vi "Read was run.vi"(8 "error in (no error)":errorcluster, 11 "WasRun in":refnum<class "WasRun.lvclass">) -> (0 "error out":errorcluster, 2 "was run":bool, 3 "WasRun out":refnum<class "WasRun.lvclass">)   [LabVIEW 2013, in "WasRun.lvclass"]
uses:
  WasRun.lvclass
  WasRun.lvclass/WasRun.ctl
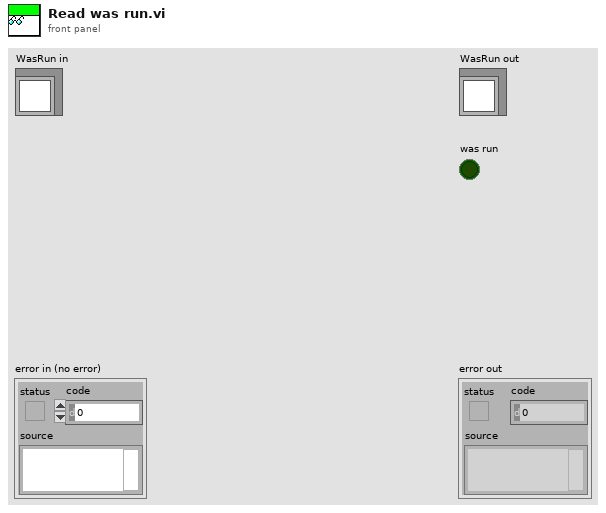
[diagram p1: front panel]
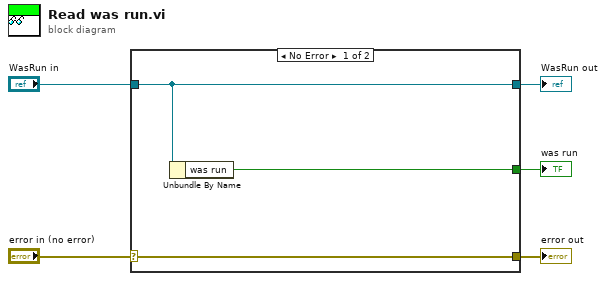
[diagram p0: block diagram]
diagram:
  n1 = case shown="No Error" "error in (no error)" {
    selector: "error in (no error)" -> [w8 w9]
    tunnel: [w8 w9] -> w4
    tunnel: [w7 w10] -> w2
    tunnel: "WasRun in" -> [w7 w10]
    tunnel: [w6 _] -> w1
    frame No Error {
      n2 = Unbundle By Name(w7) -> ("was run"=w6:bool)
    }
    frame Error {
    }
  }
  "error out" <- w4
  "WasRun out" <- w2
  "was run" <- w1
